vi "Connect Seq View Controls.vi"(8 "error in (no error)":errorcluster, 11 "teststand-api in":refnum<class "teststand-api.lvclass">) -> (0 "error out":errorcluster, 3 "teststand-api out":refnum<class "teststand-api.lvclass">)   [LabVIEW 2014, in "teststand-api.lvlib" / "teststand-api.lvclass"]
uses:
  teststand-api.lvclass
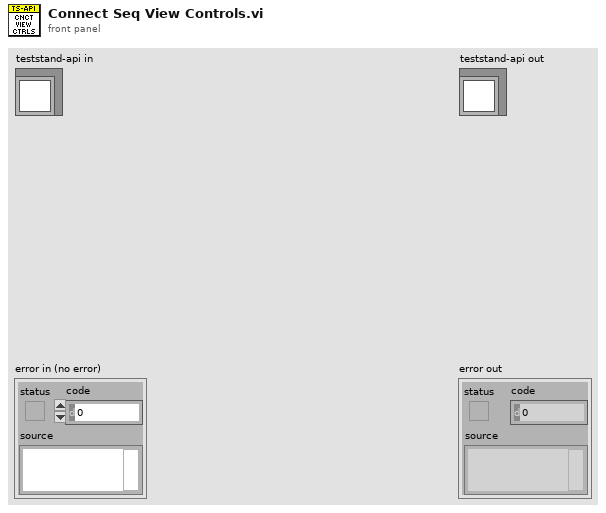
[diagram p1: front panel]
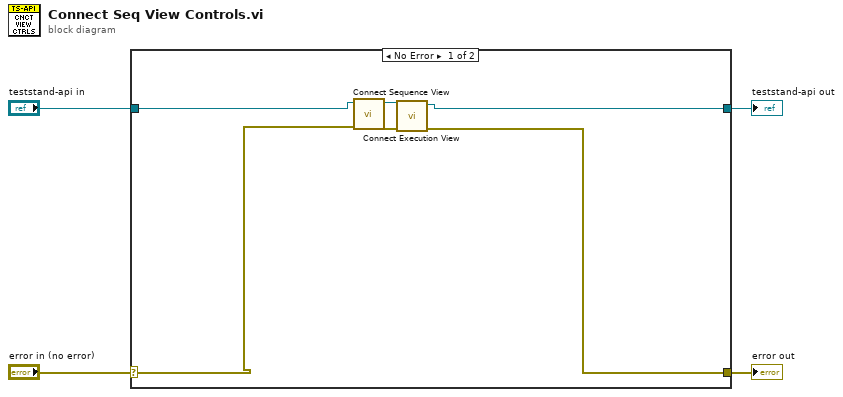
[diagram p0: block diagram]
diagram:
  n1 = case shown="No Error" "error in (no error)" {
    selector: "error in (no error)" -> [w6 w12]
    tunnel: [w5 w12] -> w3
    tunnel: [w7 w11] -> w1
    tunnel: "teststand-api in" -> [w8 w11]
    frame No Error {
      n2 = call-dynamic "Connect Sequence View.vi"("error in (no error)"=w6, "teststand-api in"=w8) -> ("error out"=w10:errorcluster, "teststand-api out"=w9:refnum<class "teststand-api.lvclass">)  [unwired: 8 in]
      n3 = call-dynamic "Connect Execution View.vi"("error in (no error)"=w10, "teststand-api in"=w9) -> ("error out"=w5:errorcluster, "teststand-api out"=w7:refnum<class "teststand-api.lvclass">)  [unwired: 8 in]
    }
    frame Error {
    }
  }
  "error out" <- w3
  "teststand-api out" <- w1
